vi "MakeSquare.vi"(8 "error in (no error)":errorcluster, 11 "KeyNumeric (Flat)":i8[](array[numeric])) -> (0 "error out":errorcluster, 3 "KeyNumeric (Square)":i8[][](array[numeric]))   [LabVIEW 2020]
uses:
  <vilib>/Utility/error.llb/Error Cluster From Error Code.vi
  <vilib>/ErrorRing/Error Ring.xnode
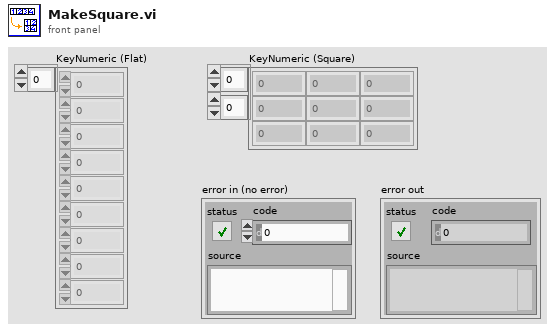
[diagram p1: front panel]
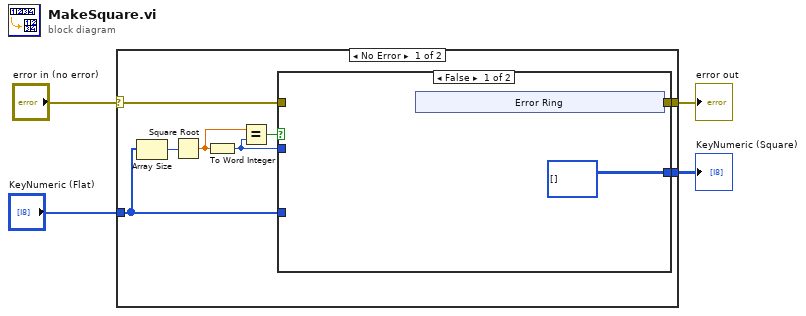
[diagram p0: block diagram]
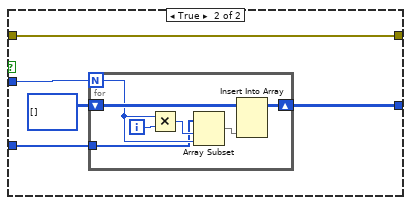
[diagram p2: hidden frame]
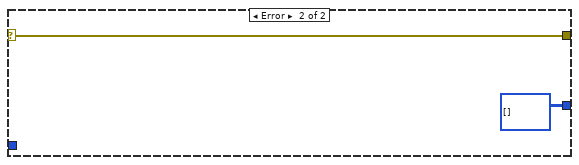
[diagram p3: hidden frame]
diagram:
  n1 = case shown="No Error" "error in (no error)" {
    selector: "error in (no error)" -> [w8 w33]
    tunnel: [w12 w33] -> w4
    tunnel: "KeyNumeric (Flat)" -> [w11 _]
    tunnel: [w9 i8[][] []] -> w2
    frame No Error {
      n2 = Array Size(array=w11) -> (size(s)=w10:i32)
      n3 = Square Root(x=w10) -> (sqrt(x)=w5:dbl)
      n4 = To Word Integer(number=w5) -> (16bit integer=w6:i16)
      n5 = Equal?(x=w5, y=w6) -> (x = y?=w7:bool)
      n6 = case shown="False" w7 {
        tunnel: w6 -> [_ w24]
        tunnel: w11 -> [_ w23]
        tunnel: w8 -> [_ w20]
        tunnel: [w14 w20] -> w12
        tunnel: [i8[][] [] w21] -> w9
        frame False {
          n7 = xnode "Error Ring"() -> ("error out"=w14:errorcluster)
        }
        frame True {
          n8 = for {
            N: w24 -> [w27]
            tunnel: w23 -> [w26]
            shift-right: [w30] -> w21
            shift-left: i8[][] [] -> [w31]
            i -> [w29]
            n9 = Multiply(x=w27, y=w29) -> (x*y=w28:i32)
            n10 = Array Subset(array=w26, index=w28, length=w27) -> (w25:i8[])
            n11 = Insert Into Array(array=w31, new element=w25) -> (w30:i8[][])  [unwired: 2 in]
          }
        }
      }
    }
    frame Error {
    }
  }
  "error out" <- w4
  "KeyNumeric (Square)" <- w2
